vi "NewControl85443091.vi"(8 "error in (no error)":errorcluster, 9 "asdf":dbl, 10 "String":string, 11 "module in":refnum<class "TesterModule.lvclass">) -> (0 "error out":errorcluster, 3 "module out":refnum<class "TesterModule.lvclass">)   [LabVIEW 2024, in "TesterModule.lvclass"]
uses:
  TesterModule.lvclass
  TesterModule.lvclass/TesterModule.ctl
  JQMHCore/Module/JQMHModule.lvclass
  NewControl85443091.ctl
  C:/DevOps/CORTEX/JQMH/JQMHCore/Module/JQMHModule.lvclass
  C:/DevOps/CORTEX/JQMH/TesterModule/TesterModule.lvclass
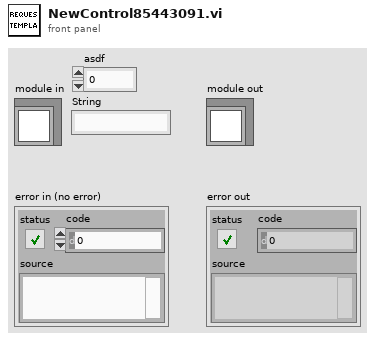
[diagram p1: front panel]
types:
  T1 = typedef "TesterModule.lvclass/NewControl85443091.ctl" = cluster{"asdf":dbl, "String":string}
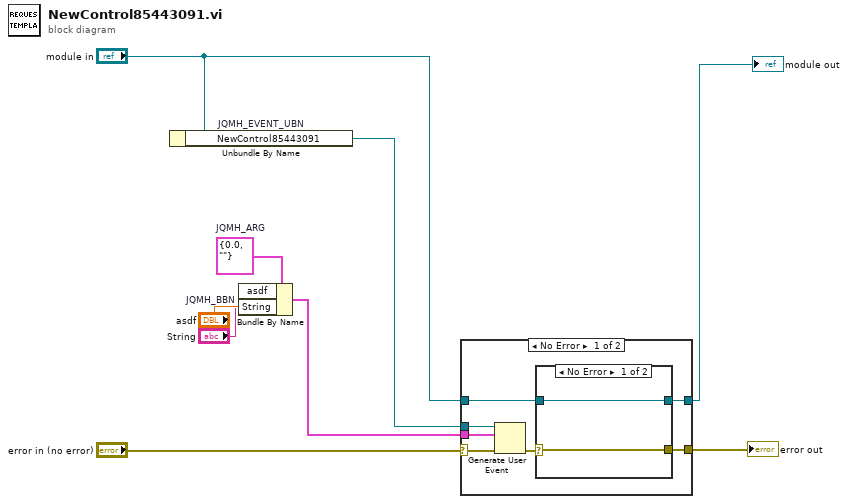
[diagram p0: block diagram]
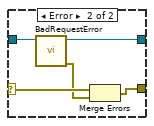
[diagram p2: hidden frame]
diagram:
  w9 = T1 {"asdf"=0.0, "String"=""}  # JQMH_ARG
  n1 = Unbundle By Name "JQMH_EVENT_UBN"("module in") -> ("NewControl85443091"=w7:refnum<user-event>)
  n2 = Bundle By Name "JQMH_BBN"(cluster=w9, "asdf"="asdf", "String"="String") -> (w8:T1)
  n3 = case shown="No Error" "error in (no error)" {
    selector: "error in (no error)" -> [w13 w24]
    tunnel: w8 -> [w16 _]
    tunnel: w7 -> [w15 _]
    tunnel: [w12 w24] -> w5
    tunnel: "module in" -> [w11 w25]
    tunnel: [w10 w25] -> w3
    frame No Error {
      n4 = Generate User Event(user event=w15, event data cluster=w16, error in=w13) -> (error out=w14:errorcluster)  [unwired: 1 in, 1 out]
      n5 = case shown="No Error" w14 {
        selector: w14 -> [w17 w23]
        tunnel: [w17 w22] -> w12
        tunnel: w11 -> [w18 w21]
        tunnel: [w18 w20] -> w10
        frame No Error {
        }
        frame Error {
          n6 = call "BadRequestError.vi"("JQMHModule in"=w21) -> ("error out"=w19:errorcluster, "JQMHModule out"=w20:refnum<class "TesterModule.lvclass">)  [unwired: 9 in]
          n7 = Merge Errors(w23, w19) -> (w22:errorcluster)
        }
      }
    }
    frame Error {
    }
  }
  "error out" <- w5
  "module out" <- w3
